vi "XYStage_Check_Status.vi"(8 "error in (no error)":errorcluster, 9 "Number of Status Tries":i32, 10 "Command/Response Cluster":T1, 11 "VISA resource name":refnum<visa-resource-name>) -> (0 "error out":errorcluster, 3 "VISA resource name out":refnum<visa-resource-name>)   [LabVIEW 2013]
panel:
  out "Non-busy Status Reply":string
  out "Status Command":string
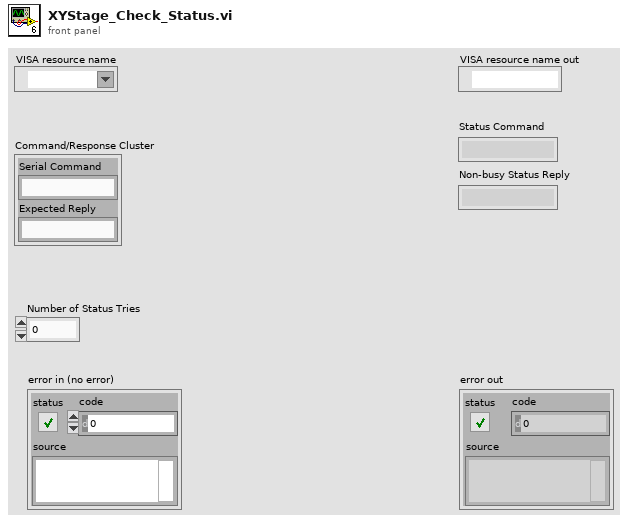
[diagram p1: front panel]
types:
  T1 = cluster{"Serial Command":string, "Expected Reply":string}
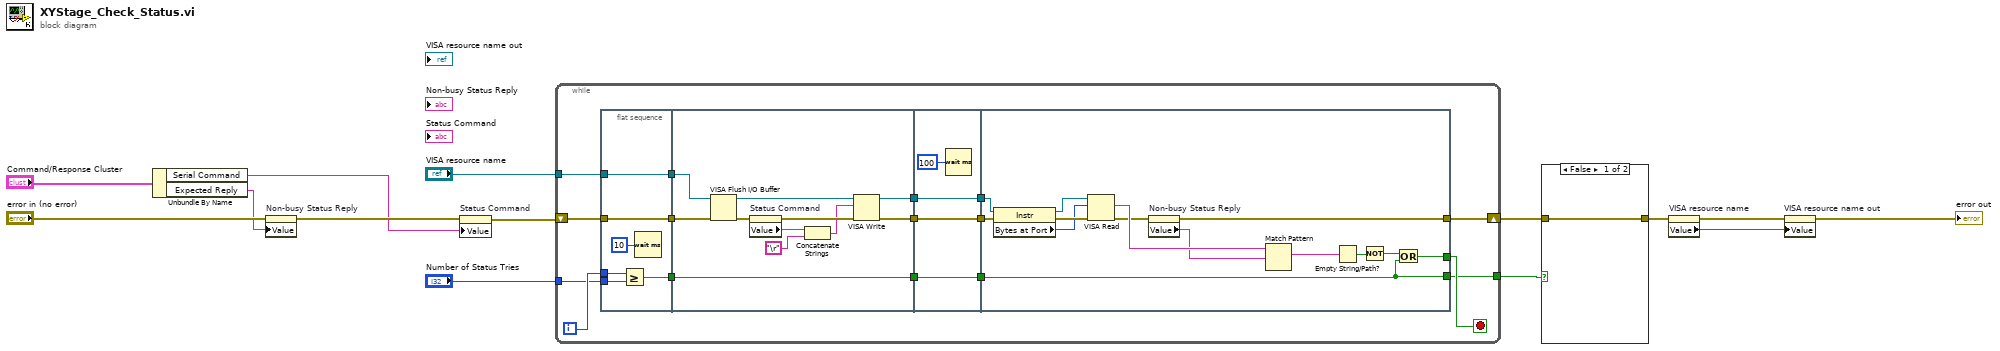
[diagram p0: block diagram]
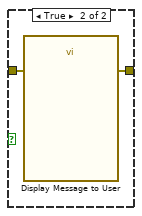
[diagram p2: hidden frame]
diagram:
  n1 = Unbundle By Name("Command/Response Cluster") -> ("Serial Command"=w3:string, "Expected Reply"=w5:string)
  n2 = property on="Non-busy Status Reply" class="Str"(error in="error in (no error)", "Value"=w5) -> (error out=w4:errorcluster)  [unwired: 1 in, 1 out]
  n3 = property on="Status Command" class="Str"(error in=w4, "Value"=w3) -> (error out=w2:errorcluster)  [unwired: 1 in, 1 out]
  n4 = while {
    tunnel: "Number of Status Tries" -> [w29]
    shift-right: [w22] -> w12
    shift-left: w2 -> [w28]
    tunnel: "VISA resource name" -> [w27]
    tunnel: [w15] -> w1
    i -> [w30]
    stop <- w23 stop-if-true
    n5 = flat-sequence {
      tunnel: w30 -> [w36]
      tunnel: w29 -> [w35]
      tunnel: w28 -> [w34]
      tunnel: w27 -> [w32]
      tunnel: [w34] -> w26
      tunnel: [w32] -> w25
      tunnel: [w31] -> w24
      tunnel: w26 -> [w47]
      tunnel: w25 -> [w46]
      tunnel: w24 -> [w37]
      tunnel: [w39] -> w21
      tunnel: [w38] -> w20
      tunnel: [w37] -> w16
      tunnel: w21 -> [w51]
      tunnel: w20 -> [w50]
      tunnel: [w51] -> w19
      tunnel: [w50] -> w18
      tunnel: [w49] -> w17
      tunnel: w16 -> [w49]
      tunnel: [w55] -> w22
      tunnel: [w53] -> w23
      tunnel: w19 -> [w58]
      tunnel: w18 -> [w57]
      tunnel: w17 -> [w52]
      tunnel: [w52] -> w15
      frame #0 {
        n6 = Greater Or Equal?(x=w36, y=w35) -> (x >= y?=w31:bool)
        n7 = Wait (ms)(milliseconds to wait=u32 10) -> ()  [unwired: 1 out]
      }
      frame #1 {
        n8 = VISA Flush I/O Buffer(VISA resource name=w46, error in (no error)=w47) -> (VISA resource name out=w43:refnum<visa-resource-name>, error out=w45:errorcluster)  [unwired: 1 in]
        n9 = property on="Status Command" class="Str"(error in=w45) -> (error out=w44:errorcluster, "Value"=w42:string)  [unwired: 1 in, 1 out]
        n10 = Concatenate Strings(w42, "\r") -> (w40:string)
        n11 = VISA Write(VISA resource name=w43, write buffer=w40, error in (no error)=w44) -> (VISA resource name out=w38:refnum<visa-resource-name>, error out=w39:errorcluster)  [unwired: 1 out]
      }
      frame #2 {
        n12 = Wait (ms)(milliseconds to wait=u32 100) -> ()  [unwired: 1 out]
      }
      frame #3 {
        n13 = property class="Instr"(reference=w57, error in=w58) -> (reference out=w61:refnum<visa-resource-name>, error out=w60:errorcluster, "Bytes at Port"=w59:u32)
        n14 = VISA Read(VISA resource name=w61, byte count=w59, error in (no error)=w60) -> (read buffer=w65:string, error out=w56:errorcluster)  [unwired: 2 out]
        n15 = property on="Non-busy Status Reply" class="Str"(error in=w56) -> (error out=w55:errorcluster, "Value"=w54:string)  [unwired: 1 in, 1 out]
        n16 = Match Pattern(string=w65, regular expression=w54) -> (match substring=w64:string)  [unwired: 1 in, 3 out]
        n17 = Empty String/Path?(string/path=w64) -> (empty?=w63:bool)
        n18 = Not(x=w63) -> (.not. x?=w62:bool)
        n19 = Or(x=w62, y=w52) -> (x .or. y?=w53:bool)
      }
    }
  }
  n20 = case shown="False" w1 {
    tunnel: w12 -> [w66 w68]
    tunnel: [w66 w67] -> w9
    frame False {
    }
    frame True {
      n21 = call "Display Message to User"("error in (no error)"=w68) -> ("error out"=w67:errorcluster)  [unwired: 9 in, 1 out]
    }
  }
  n22 = property on="VISA resource name" class="VISAName"(error in=w9) -> (error out=w10:errorcluster, "Value"=w11:refnum<visa-resource-name>)  [unwired: 1 in, 1 out]
  n23 = property on="VISA resource name out" class="VISAName"(error in=w10, "Value"=w11) -> (error out=→"error out":errorcluster)  [unwired: 1 in, 1 out]
